vi "IPC-Core-MainModule.vi"(0 "CmdQRef":refnum<queue>, 1 "ModbusQRef":refnum<queue>, 2 "DaqQRef":refnum<queue>, 3 "UdpQRef":refnum<queue>, 4 "ErrorQRef":refnum<queue>, 5 "error in":errorcluster) -> (19 "error out":errorcluster)   [LabVIEW 2014]
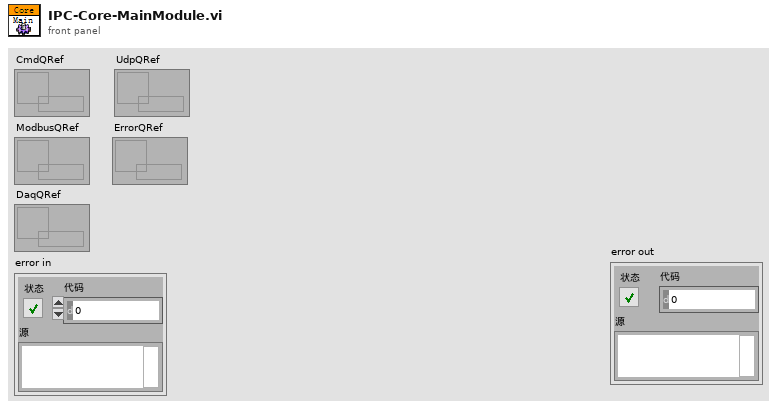
[diagram p1: front panel]
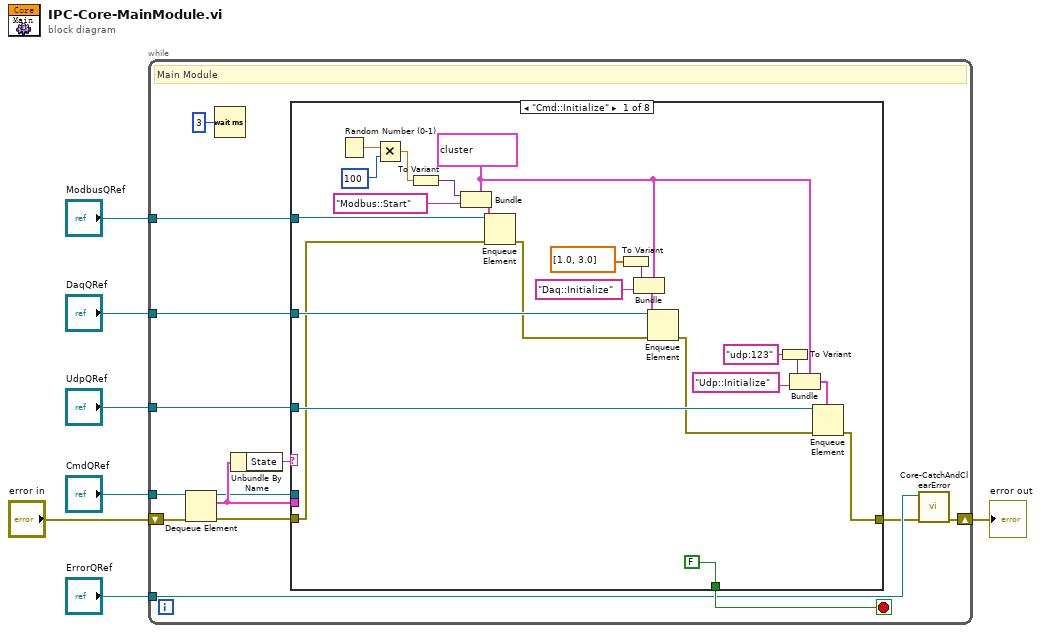
[diagram p0: block diagram]
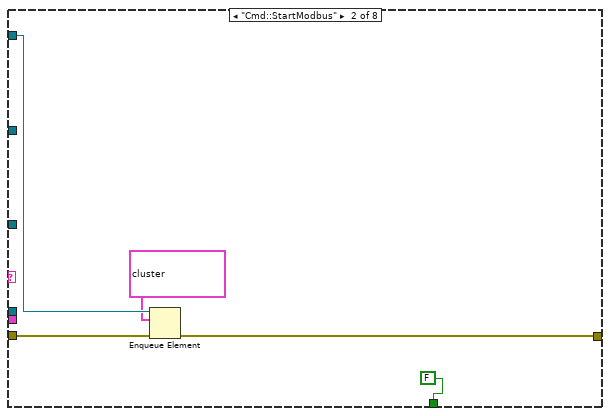
[diagram p2: hidden frame]
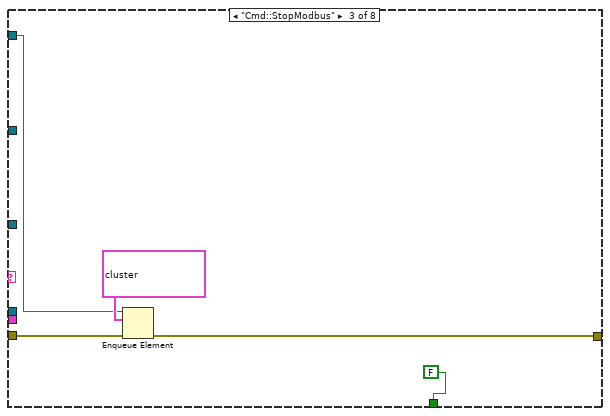
[diagram p3: hidden frame]
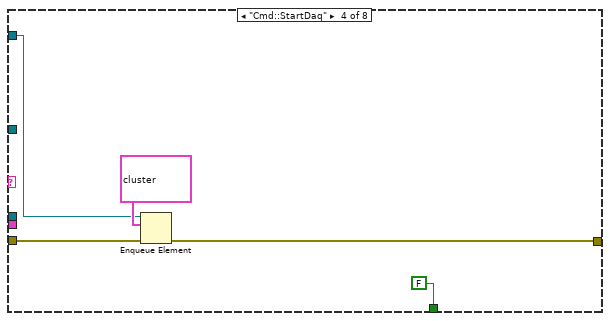
[diagram p4: hidden frame]
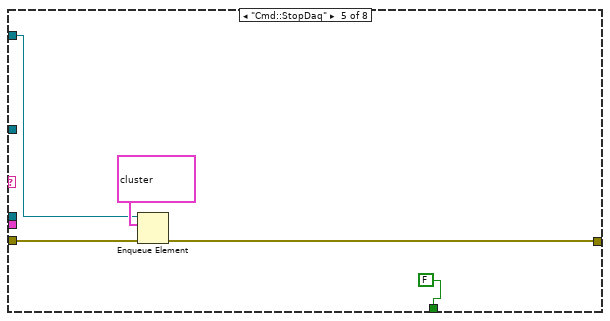
[diagram p5: hidden frame]
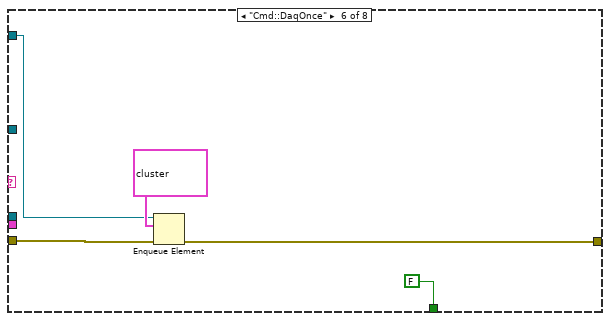
[diagram p6: hidden frame]
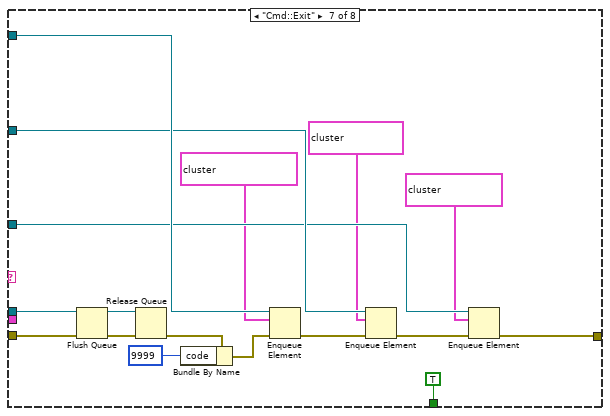
[diagram p7: hidden frame]
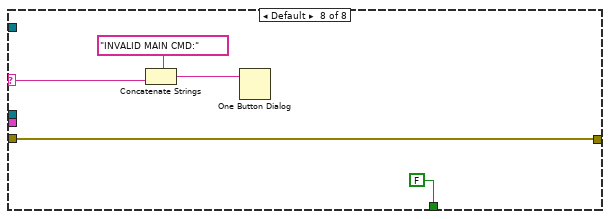
[diagram p8: hidden frame]
diagram:
  n1 = while {
    tunnel: "CmdQRef" -> [w21]
    shift-right: [w8] -> w1
    shift-left: "error in" -> [w20]
    tunnel: "ErrorQRef" -> [w10]
    tunnel: "ModbusQRef" -> [w15]
    tunnel: "DaqQRef" -> [w14]
    tunnel: "UdpQRef" -> [w13]
    stop <- w11 stop-if-true
    # "Main Module"
    n2 = Dequeue Element(queue=w21, error in (no error)=w20) -> (queue out=w12:refnum<queue>, element=w16:cluster{"Data":variant, "State":string}, error out=w19:errorcluster)  [unwired: 1 in, 1 out]
    n3 = Wait (ms)(milliseconds to wait=u32 3 ("等待时间（毫秒）")) -> ()  [unwired: 1 out]
    n4 = Unbundle By Name(w16) -> ("State"=w18:string)
    n5 = case shown="\"Cmd::Initialize\"" w18 {
      selector: w18 -> [_ _ _ _ _ _ _ w90]
      tunnel: w19 -> [w25 w48 w53 w56 w62 w65 w84 w91]
      tunnel: [w22 w47 w51 w57 w63 w67 w76 w91] -> w9
      tunnel: w16 -> [_ _ _ _ _ _ _ _]
      tunnel: w15 -> [w37 w49 w52 _ _ _ w75 _]
      tunnel: w14 -> [w36 _ _ w55 w61 w68 w74 _]
      tunnel: w13 -> [w35 _ _ _ _ _ w73 _]
      tunnel: w12 -> [_ _ _ _ _ _ w83 _]
      tunnel: [FALSE FALSE FALSE FALSE FALSE FALSE TRUE FALSE] -> w11
      frame "Cmd::Initialize" {
        w26 = cluster{"Data":variant, "State":string} {"Data"=variant, "State"=""}
        n6 = Random Number (0-1)() -> (number: 0 to 1=w29:dbl)
        n7 = Multiply(x=w29, y=100) -> (x*y=w27:dbl)
        n8 = To Variant(anything=w27) -> (Variant=w39:variant)
        n9 = Bundle(cluster=w26, "Data"=w39, "State"="Modbus::Start") -> (w44:cluster{"Data":variant, "State":string})
        n10 = Enqueue Element(queue=w37, element=w44, error in (no error)=w25) -> (error out=w24:errorcluster)  [unwired: 1 in, 2 out]
        n11 = To Variant(anything=dbl[] [1.0, 3.0]) -> (Variant=w40:variant)
        n12 = Bundle(cluster=w26, "Data"=w40, "State"="Daq::Initialize") -> (w42:cluster{"Data":variant, "State":string})
        n13 = Enqueue Element(queue=w36, element=w42, error in (no error)=w24) -> (error out=w23:errorcluster)  [unwired: 1 in, 2 out]
        n14 = To Variant(anything="udp:123") -> (Variant=w32:variant)
        n15 = Bundle(cluster=w26, "Data"=w32, "State"="Udp::Initialize") -> (w31:cluster{"Data":variant, "State":string})
        n16 = Enqueue Element(queue=w35, element=w31, error in (no error)=w23) -> (error out=w22:errorcluster)  [unwired: 1 in, 2 out]
      }
      frame "Cmd::StartModbus" {
        n17 = Enqueue Element(queue=w49, element=cluster{"Data":variant, "State":string} {"Data"=variant, "State"="Modbus::Start"} ("元素"), error in (no error)=w48) -> (error out=w47:errorcluster)  [unwired: 1 in, 2 out]
      }
      frame "Cmd::StopModbus" {
        n18 = Enqueue Element(queue=w52, element=cluster{"Data":variant, "State":string} {"Data"=variant, "State"="Modbus::Pause"} ("元素"), error in (no error)=w53) -> (error out=w51:errorcluster)  [unwired: 1 in, 2 out]
      }
      frame "Cmd::StartDaq" {
        n19 = Enqueue Element(queue=w55, element=cluster{"Data":variant, "State":string} {"Data"=variant, "State"="Daq::Start"} ("元素"), error in (no error)=w56) -> (error out=w57:errorcluster)  [unwired: 1 in, 2 out]
      }
      frame "Cmd::StopDaq" {
        n20 = Enqueue Element(queue=w61, element=cluster{"Data":variant, "State":string} {"Data"=variant, "State"="Daq::Pause"} ("元素"), error in (no error)=w62) -> (error out=w63:errorcluster)  [unwired: 1 in, 2 out]
      }
      frame "Cmd::DaqOnce" {
        n21 = Enqueue Element(queue=w68, element=cluster{"Data":variant, "State":string} {"Data"=variant, "State"="Daq::Once"} ("元素"), error in (no error)=w65) -> (error out=w67:errorcluster)  [unwired: 1 in, 2 out]
      }
      frame "Cmd::Exit" {
        n22 = Flush Queue(queue=w83, error in (no error)=w84) -> (queue out=w86:refnum<queue>, error out=w85:errorcluster)  [unwired: 1 out]
        n23 = Release Queue(queue=w86, error in (no error)=w85) -> (error out=w81:errorcluster)  [unwired: 1 in, 2 out]
        n24 = Bundle By Name(cluster=w81, "code"=9999) -> (w79:errorcluster)
        n25 = Enqueue Element(queue=w75, element=cluster{"Data":variant, "State":string} {"Data"=variant, "State"="Modbus::Exit"}, error in (no error)=w79) -> (error out=w78:errorcluster)  [unwired: 1 in, 2 out]
        n26 = Enqueue Element(queue=w74, element=cluster{"Data":variant, "State":string} {"Data"=variant, "State"="Daq::Exit"}, error in (no error)=w78) -> (error out=w77:errorcluster)  [unwired: 1 in, 2 out]
        n27 = Enqueue Element(queue=w73, element=cluster{"Data":variant, "State":string} {"Data"=variant, "State"="Udp::Exit"}, error in (no error)=w77) -> (error out=w76:errorcluster)  [unwired: 1 in, 2 out]
      }
      frame Default {
        n28 = Concatenate Strings("INVALID MAIN CMD:", w90) -> (w88:string)
        n29 = One Button Dialog(message=w88) -> ()  [unwired: 1 in, 1 out]
      }
    }
    n30 = call "Core-CatchAndClearError.vi"("error in (no error)"=w9, "ErrorQ"=w10) -> ("error out"=w8:errorcluster)  [unwired: 7 in]
  }
  "error out" <- w1
